vi "lm Assign LE Colors.vi"(8 "error in (no error)":errorcluster, 11 "strColorArray":string) -> (0 "error out":errorcluster, 2 "function return":i32, 3 "strColorArray out":string)   [LabVIEW 2015, in "LumencorDLL32.lvlib"]
doc: "extern \"C\" LUMENCORDLL2B_API int lmAssignLEColors(char *strColorArray);"
uses:
  <userlib>/LumencorDLL32/LumencorDLL32.lvlib
  <userlib>/LumencorDLL32/LumencorDLL32.dll
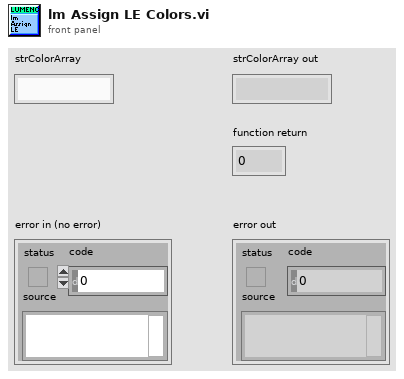
[diagram p1: front panel]
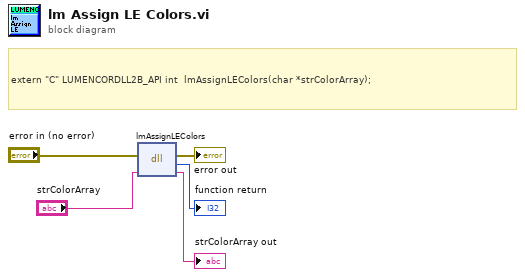
[diagram p0: block diagram]
diagram:
  # "extern \"C\" LUMENCORDLL2B_API int  lmAssignLEColors(char *strColorArray);"
  n1 = dll-call lib="C:/Program Files (x86)/National Instruments/LabVIEW 2015/user.lib/LumencorDLL32/LumencorDLL32.*" fn="lmAssignLEColors"(error in="error in (no error)", "strColorArray"="strColorArray") -> (error out=→"error out":errorcluster, →"function return":i32, "strColorArray"=→"strColorArray out":string)  [unwired: 2 in, 1 out]
